vi "Query Movement.vi"(8 "error in (no error)":errorcluster, 10 "Motor ID (0)":u8, 11 "VISA resource name":refnum<visa-resource-name>) -> (0 "error out":errorcluster, 2 "Motor Moving":bool, 3 "VISA resource name out":refnum<visa-resource-name>)   [LabVIEW 2016, in "Dynamixel Motor.lvlib"]
doc: "Checks to see if the motor is attempting to reach its goal position."
uses:
  Dynamixel Motor.lvlib
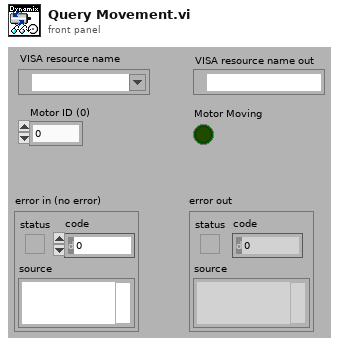
[diagram p1: front panel]
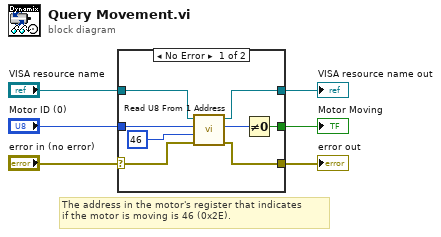
[diagram p0: block diagram]
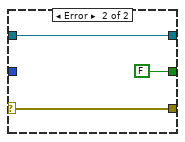
[diagram p2: hidden frame]
diagram:
  # "The address in the motor's register that indicates \nif the motor is moving is 46 (0x2E)."
  n1 = case shown="No Error" "error in (no error)" {
    selector: "error in (no error)" -> [w7 w16]
    tunnel: [w13 FALSE] -> w6
    tunnel: "VISA resource name" -> [w12 w17]
    tunnel: [w11 w17] -> w4
    tunnel: [w10 w16] -> w3
    tunnel: "Motor ID (0)" -> [w9 _]
    frame No Error {
      n2 = call "Read U8 From 1 Address.vi"("Error in (no error)"=w7, "Address number (0)"=u8 46 ("Address # DEC"), "Motor ID (0)"=w9, "VISA resource name"=w12) -> ("error out"=w10:errorcluster, "Data"=w14:u8, "VISA resource name out"=w11:refnum<visa-resource-name>)  [unwired: 5 in]
      n3 = Not Equal To 0?(x=w14) -> (x != 0?=w13:bool)
    }
    frame Error {
    }
  }
  "VISA resource name out" <- w4
  "error out" <- w3
  "Motor Moving" <- w6
